vi "daqCreateFile.vi"   [LabVIEW 2017]
uses:
  globalUtilities.vi
  globalDevices.vi
types:
  T1 = enum16{"open", "replace", "create", "open or create", "replace or create", "replace or create with confirmation"}
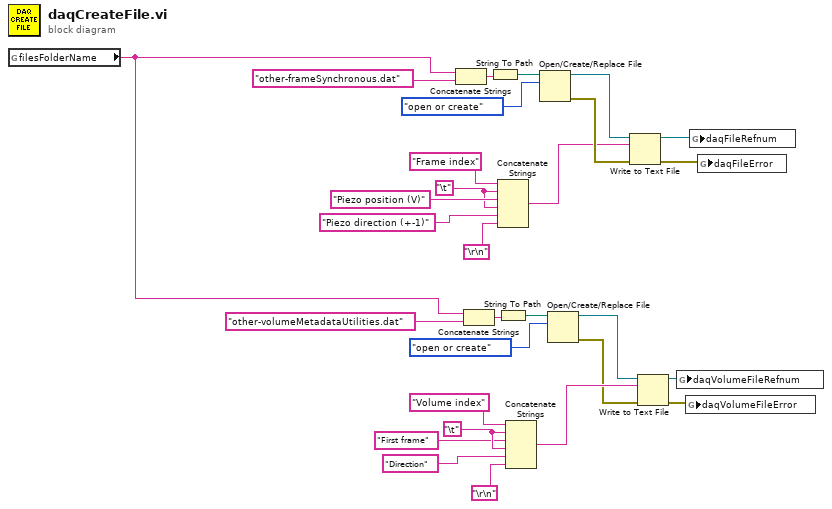
[diagram p0: block diagram]
diagram:
  w11 = "\t"
  w20 = "\t"
  n1 = global read "globalUtilities.vi" "filesFolderName"() -> (w1:string)
  n2 = Concatenate Strings(w1, "other-frameSynchronous.dat") -> (w28:string)
  n3 = Concatenate Strings(w1, "other-volumeMetadataUtilities.dat") -> (w3:string)
  n4 = String To Path(string=w28) -> (path=w27:path)
  n5 = Concatenate Strings("Frame index" ("string"), w20, "Piezo position (V)" ("string"), w20, "Piezo direction (+-1)" ("string"), "\r\n") -> (w21:string)
  n6 = String To Path(string=w3) -> (path=w4:path)
  n7 = Concatenate Strings("Volume index" ("string"), w11, "First frame" ("string"), w11, "Direction" ("string"), "\r\n") -> (w10:string)
  n8 = Open/Create/Replace File(file path (use dialog)=w27, operation (0:open)=T1."open or create") -> (refnum out=w25:refnum<file>, error out=w24:errorcluster)  [unwired: 4 in, 1 out]
  n9 = Open/Create/Replace File(file path (use dialog)=w4, operation (0:open)=T1."open or create") -> (refnum out=w6:refnum<file>, error out=w7:errorcluster)  [unwired: 4 in, 1 out]
  n10 = Write to Text File(file (use dialog)=w25, text=w21, error in=w24) -> (refnum out=w17:refnum<file>, error out=w16:errorcluster)  [unwired: 1 in, 1 out]
  n11 = Write to Text File(file (use dialog)=w6, text=w10, error in=w7) -> (refnum out=w14:refnum<file>, error out=w15:errorcluster)  [unwired: 1 in, 1 out]
  n12 = global write "globalDevices.vi" "daqVolumeFileRefnum"(w14) -> ()
  n13 = global write "globalDevices.vi" "daqVolumeFileError"(w15) -> ()
  n14 = global write "globalDevices.vi" "daqFileRefnum"(w17) -> ()
  n15 = global write "globalDevices.vi" "daqFileError"(w16) -> ()
